vi "number-in-counts-k1.vi"(8 "error in (no error)":errorcluster, 9 "unit":enum16{"fs", "ps", "um", "mm", "counts"}(ring), 11 "Number":dbl) -> (0 "error out":errorcluster, 2 "counts":dbl format="%#_18f")   [LabVIEW 2009]
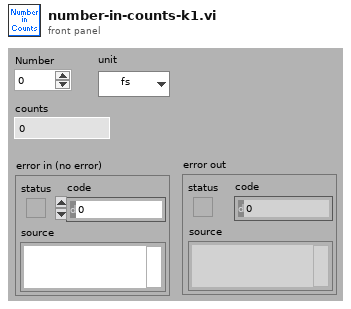
[diagram p1: front panel]
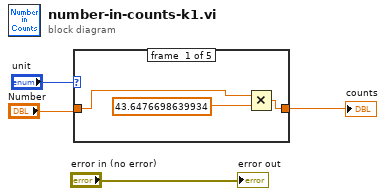
[diagram p0: block diagram]
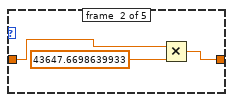
[diagram p2: hidden frame]
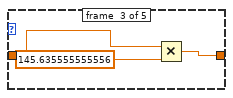
[diagram p3: hidden frame]
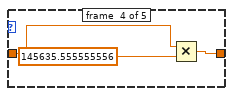
[diagram p4: hidden frame]
diagram:
  n1 = case shown="\"fs\", Default" "unit" {
    tunnel: "Number" -> [w5 w8 w11 w14 w17]
    tunnel: [w7 w10 w13 w16 w17] -> w2
    frame #0 {
      n2 = Multiply(x=w5, y=43.6476698639934) -> (x*y=w7:dbl)
    }
    frame #1 {
      n3 = Multiply(x=w8, y=43647.6698639933) -> (x*y=w10:dbl)
    }
    frame #2 {
      n4 = Multiply(x=w11, y=145.635555555556) -> (x*y=w13:dbl)
    }
    frame #3 {
      n5 = Multiply(x=w14, y=145635.555555556) -> (x*y=w16:dbl)
    }
    frame #4 {
    }
  }
  "counts" <- w2
  "error out" <- "error in (no error)"
